vi "Format Toggle Key Cell.vi"(8 "Error in":errorcluster caption="Error in (no error)", 11 "ToggleKeyBind":T1) -> (0 "Error out":errorcluster, 3 "Toggle Key Text":string)   [LabVIEW 2023, in "VIDoc Printer.lvlib" / "VIDoc Printer.lvclass"]
doc: "Converts the Toggle Key Bind information into a printable String."
uses:
  VIDoc Printer.lvclass
  <vilib>/Utility/miscctls.llb/LVKeyTypeDef.ctl
  VIDoc Printer.lvclass/VIDoc Printer.ctl
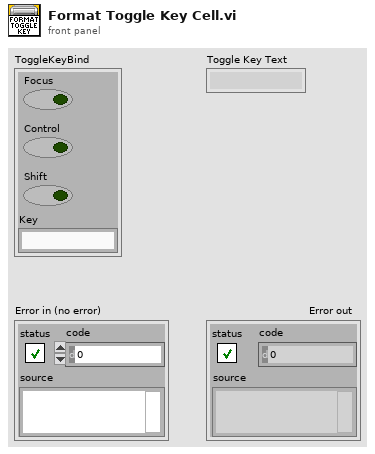
[diagram p1: front panel]
types:
  T1 = typedef "LVKeyTypeDef.ctl" = cluster{"Focus":bool, "Control":bool, "Shift":bool, "Key":string}
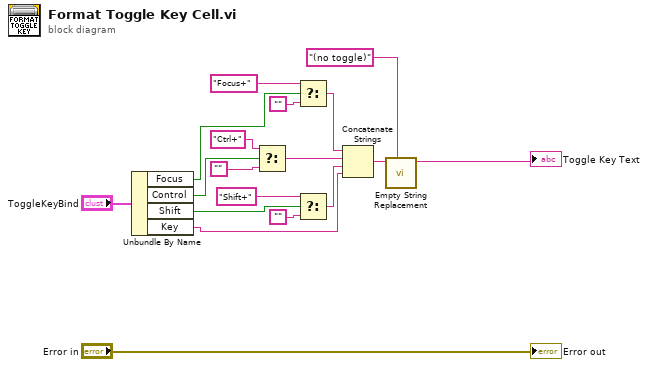
[diagram p0: block diagram]
diagram:
  n1 = Unbundle By Name("ToggleKeyBind") -> ("Focus"=w15:bool, "Control"=w10:bool, "Shift"=w5:bool, "Key"=w16:string)
  n2 = Select(t="Ctrl+" ("String"), s=w10, f="") -> (s? t:f=w8:string)
  n3 = Select(t="Focus+" ("String"), s=w15, f="") -> (s? t:f=w12:string)
  n4 = Select(t="Shift+" ("String"), s=w5, f="") -> (s? t:f=w4:string)
  n5 = Concatenate Strings(w12, w8, w4, w16) -> (w3:string)
  n6 = call "Empty String Replacement.vi"("Empty"="(no toggle)", "String"=w3) -> ("String Out"=→"Toggle Key Text":string)  [unwired: 9 in]
  "Error out" <- "Error in"
